vi "Main modul map v3.vi"() -> ()   [LabVIEW 2012]
uses:
  <vilib>/Utility/miscctls.llb/LVPoint32TypeDef.ctl
  <vilib>/addons/Fuzzy Logic/FL Fuzzy Controller (MIMO).vi
  Matematyczne/Matematyczne.lvlib
  <vilib>/addons/Fuzzy Logic/NI_Fuzzy_Logic_API.lvlib
panel:
  out "String":string
  in  "zad. promien odlegl.":dbl
  in  "Autonomia":bool
  out "Azymut [stopnie]":dbl
  out "Lista współrzędnych":string[][](table)
  in  "Ostatni zaznaczony punkt na mapie":cluster{"X":i32, "Y":i32}
  in  "Pocz. poł. \nrobota":T1={"UTM"={"E [m]"=393271.81, "N [m]"=5734673.27, "Strefa"=""}, "Poł. startowe"={"Piksel x"=0, "Piksel y"=0}} caption="Początkowe położenie robota" {"UTM"."N [m]" format="%#_10g"}
  in  "Tab Control":T2(tab)
  in  "Tryb GPS / Kin":u16(ring) caption="Dane na podstawie których ma działać mapa" items=["Współrzędne geografczne", "Kinematyka robota"]
  in  "Azymut robota":dbl
  in  "Lokalizacja mapy terenu":path=path "C:/Users/User/Desktop/pł.JPG"
  in  "Parametry odwzorowania Ziemi (WGS84)":cluster{"a":dbl, "b":dbl}={"a"=6378137.0, "b"=6356752.3142} {"b" format="%#.6g"; "a" format="%#.6g"}
  in  "Współrzędne geograficzne 2":string
  in  "Wyznaczanie odległości":T3(ring)=enum."Odległość pomiędzy znacznikami"
  in  "Współrzędne geograficzne 1":string
  in  "Blokada \nznaczników":bool
  in  "Zatwierdz ustalony zakres":bool
  in  "Kolor  znaczników":u32(colorbox)=16774930
  in  "Polozenie 2":cluster{"X":i32, "Y":i32}={"X"=358, "Y"=265}
  in  "Polozenie 1":cluster{"X":i32, "Y":i32}={"X"=265, "Y"=265}
  in  "Położenie na mapie":bool
  in  "Wybór \nznacznika":bool
  in  "Zaznaczona\n odleglość [m]":dbl=15.0
  in  "Zakres skali":u16(ring)=11 items=["do 1m", "do 5m", "do 10m", "do 50m", "do 100m", "do 200m", "do 500m", "do 1km", "do 5km", "do 10km", "Dubai", "OSM 10m", "OSM 30m", "OSM 50m", "OSM 100m"]
  in  "Grubość \nznaczników":u32=2
  in  "Nazwa":string
  in  "Współrzędna punktu":string
  in  "Dodaj punkt wsp.":bool
  in  "Dodaj punkt odl.":bool
  in  "Odleglosc do\n zaznaczonego punktu [m]":cluster{"X":dbl, "Y":dbl} caption="Odleglosc do zaznaczonego punktu [m] od startu"
  in  "Nazwa zaznaczonego punktu":string
  in  "Punkt do usunięcia":u16(ring) items=[""=1, "B"=2, "B"=3, "B"=4, "B"=5, "C"=6, "D"=7]
  in  "Usuń punkt":bool
  in  "Wyczyść trasę":bool
  in  "Położenie startu":bool
  in  "Kierunek na punkt":u16(ring) items=[""=1, "B"=2, "B"=3, "B"=4, "B"=5, "C"=6, "D"=7]
  out "Położenie \nrobota  UTM":T4 {"E [m]" format="%#_10g"; "N [m]" format="%#_12g"}
  out "Szerokośc geograficzna - GPS":dbl format="%_9f"
  out "Długość geograficzna - GPS":dbl format="%_9f"
  in  "Centrowanie położenia":bool
  in  "Azymut":dbl
  out "Kierunek":picture
  in  "Początkowe położenie robota":u32(colorbox)=15663118
  in  "Trasa robota":u32(colorbox)
  in  "Kierunek ruchu robota":u32(colorbox)=15663118
  in  "Zoom mapy":sgl(slide)=1.0 scale=0.2..4.0
  in  "Układ współrzędnych":u32(colorbox)
  in  "Zaznaczony punkt":u32(colorbox)=15663118 caption="Ostatni zaznaczony punkt kursorem"
  in  "Wpisane punkty na\nliście współrzędnych":u32(colorbox)=12271
  in  "Mouse down coords":T5
  out "Mapa":picture caption="Mapa z wprowadzonym punktem"
  in  "stop":bool
  # "Ustawienia dla danych z GPS\nPodstaowe parametry Ziemi dla układu WGS84"
  # "Ustawienia dla kinematyki robota."
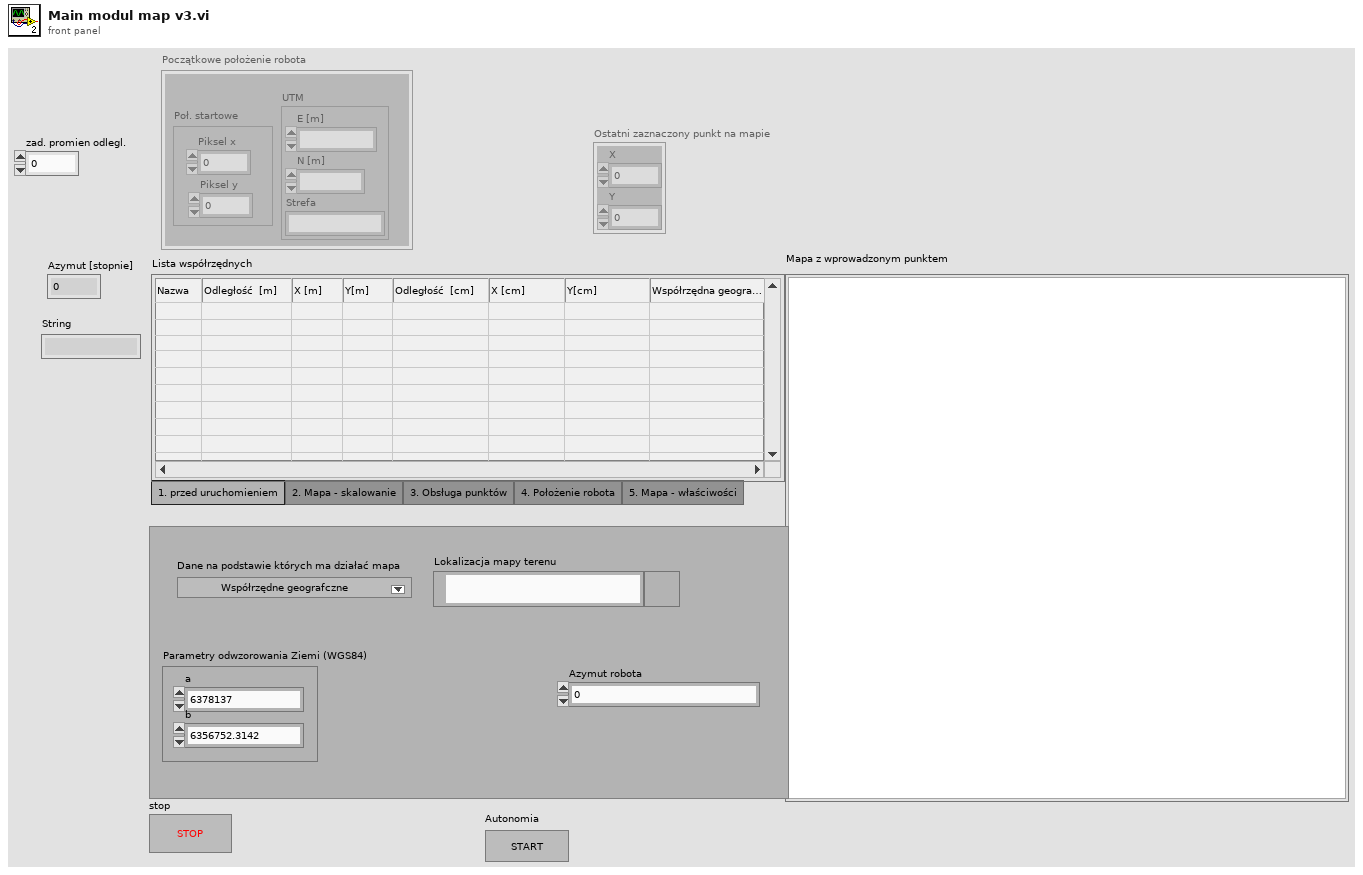
[diagram p1: front panel]
types:
  T1 = cluster{"UTM":cluster{"E [m]":ext, "N [m]":ext, "Strefa":string}, "Poł. startowe":cluster{"Piksel x":i32, "Piksel y":i32}}
  T2 = enum32{"1. przed uruchomieniem", "2. Mapa - skalowanie", "3. Obsługa punktów", "4. Położenie robota", "5. Mapa - właściwości"}
  T3 = enum16{"Współrzędne geograficzne", "Odległość pomiędzy znacznikami"}
  T4 = cluster{"E [m]":ext, "N [m]":ext, "Strefa":string}
  T5 = typedef "LVPoint32TypeDef.ctl" = cluster{"Horizontal":i32, "Vertical":i32}
  T6 = cluster{"Przesunięcie mapy":cluster{"X":i16, "Y":i16}, "Zoom":dbl, "Długość piksela w metrach":dbl}
  T7 = enum16{"Pobranie punktu", "Obrót i dojazd do punktu", "Zatrzymanie w punkcie", "Powrót na start"}
  T8 = typedef "NI_Fuzzy_Logic_API.lvlib/FL System.ctl" = cluster{"input variables":T9[], "output variables":T9[], "rules":T12[], "defuzzification method":T18, "description":string, "user MF interpolating polynomials":T19[]}
  T9 = typedef "NI_Fuzzy_Logic_API.lvlib/FL Variable.ctl" = cluster{"name":string, "range":dbl[], "MFs":T10[]}
  T10 = typedef "NI_Fuzzy_Logic_API.lvlib/FL Membership Function.ctl" = cluster{"name":string, "shape":T11, "points":dbl[], "color":u32, "user-defined shape index":i32}
  T11 = typedef "NI_Fuzzy_Logic_API.lvlib/FL Membership Function Shape.ctl" = u16
  T12 = typedef "NI_Fuzzy_Logic_API.lvlib/FL Rule.ctl" = cluster{"antecedents":T13[], "antecedent connective":T15, "consequents":T16[], "consequent implication":T17, "degree of support":dbl}
  T13 = typedef "NI_Fuzzy_Logic_API.lvlib/FL Antecedent.ctl" = cluster{"Var Index":i32, "MF Index":i32, "Cond":T14}
  T14 = typedef "NI_Fuzzy_Logic_API.lvlib/FL Modifier.ctl" = u16
  T15 = typedef "NI_Fuzzy_Logic_API.lvlib/FL Antecedent Connective.ctl" = u16
  T16 = typedef "NI_Fuzzy_Logic_API.lvlib/FL Consequent.ctl" = cluster{"Var Index":i32, "MF Index":i32, "Cond":T14}
  T17 = typedef "NI_Fuzzy_Logic_API.lvlib/FL Consequent Implication.ctl" = u16
  T18 = typedef "NI_Fuzzy_Logic_API.lvlib/FL Defuzzification.ctl" = u16
  T19 = typedef "NI_Fuzzy_Logic_API.lvlib/FL Interpolating polynomials.ctl" = cluster{"X":dbl[], "Y":dbl[], "Y(x) coeff":dbl[][], "X(y) coeff":dbl[][], "Area(y) coeff":dbl[][], "coa_x(y) coeff":dbl[][]}
  T20 = cluster{"Położenie grotu":cluster{"Pixel x":i16, "Pixel y":i16}, "Kolor":u32, "Długość [px]":u32, "Kąt/azymut":dbl, "Interpretacją kąta ustawienia strzałki":enum16{"Kąt trygonometryczny", "Azymut"}, "Grubość":u32, "Długość grotu":u32}
  T21 = cluster{"Położenie  środka":cluster{"Pixel x":i16, "Pixel y":i16}, "Kolor ":u32, "Grubość  ":u32}
  T22 = cluster{"Położenie":cluster{"Pixel x":i16, "Pixel y":i16}, "Kolor punktu":u32, "Rozmiar punktu":u32, "Nazwa punktu":string}
  T23 = cluster{"Kolor punktów z listy":u32, "Położenie startowe robota":cluster{"Pixel y":i16, "Pixel x":i16}}
  T24 = cluster{"Kolor skali":u32, "Odległość siatki od startu":cluster{"X [m]":dbl, "Y [m]":dbl}, "Poł. startowe":cluster{"Piksel x":i32, "Piksel y":i32}}
  T25 = cluster{"Nazwa zaznaczonego punktu":string, "Odleglosc do\n zaznaczonego punktu [m]":cluster{"X":dbl, "Y":dbl}}
  T26 = cluster{"UTM":cluster{"E_coord[m]":ext, "N_coord[m]":ext, "Strefa":string}, "Poł. startowe":cluster{"Piksel x":i32, "Piksel y":i32}}
  T27 = typedef "LVBoundsTypeDef.ctl" = cluster{"Width":u32, "Height":u32}
  T28 = typedef "LVMouseTypeDef.ctl" = cluster{"Mouse Position":cluster{"X":i32, "Y":i32}, "Mouse Modifiers":cluster{"Button Down":bool, "Shift Mod":bool, "Menu Mod":bool, "Option Mod":bool}}
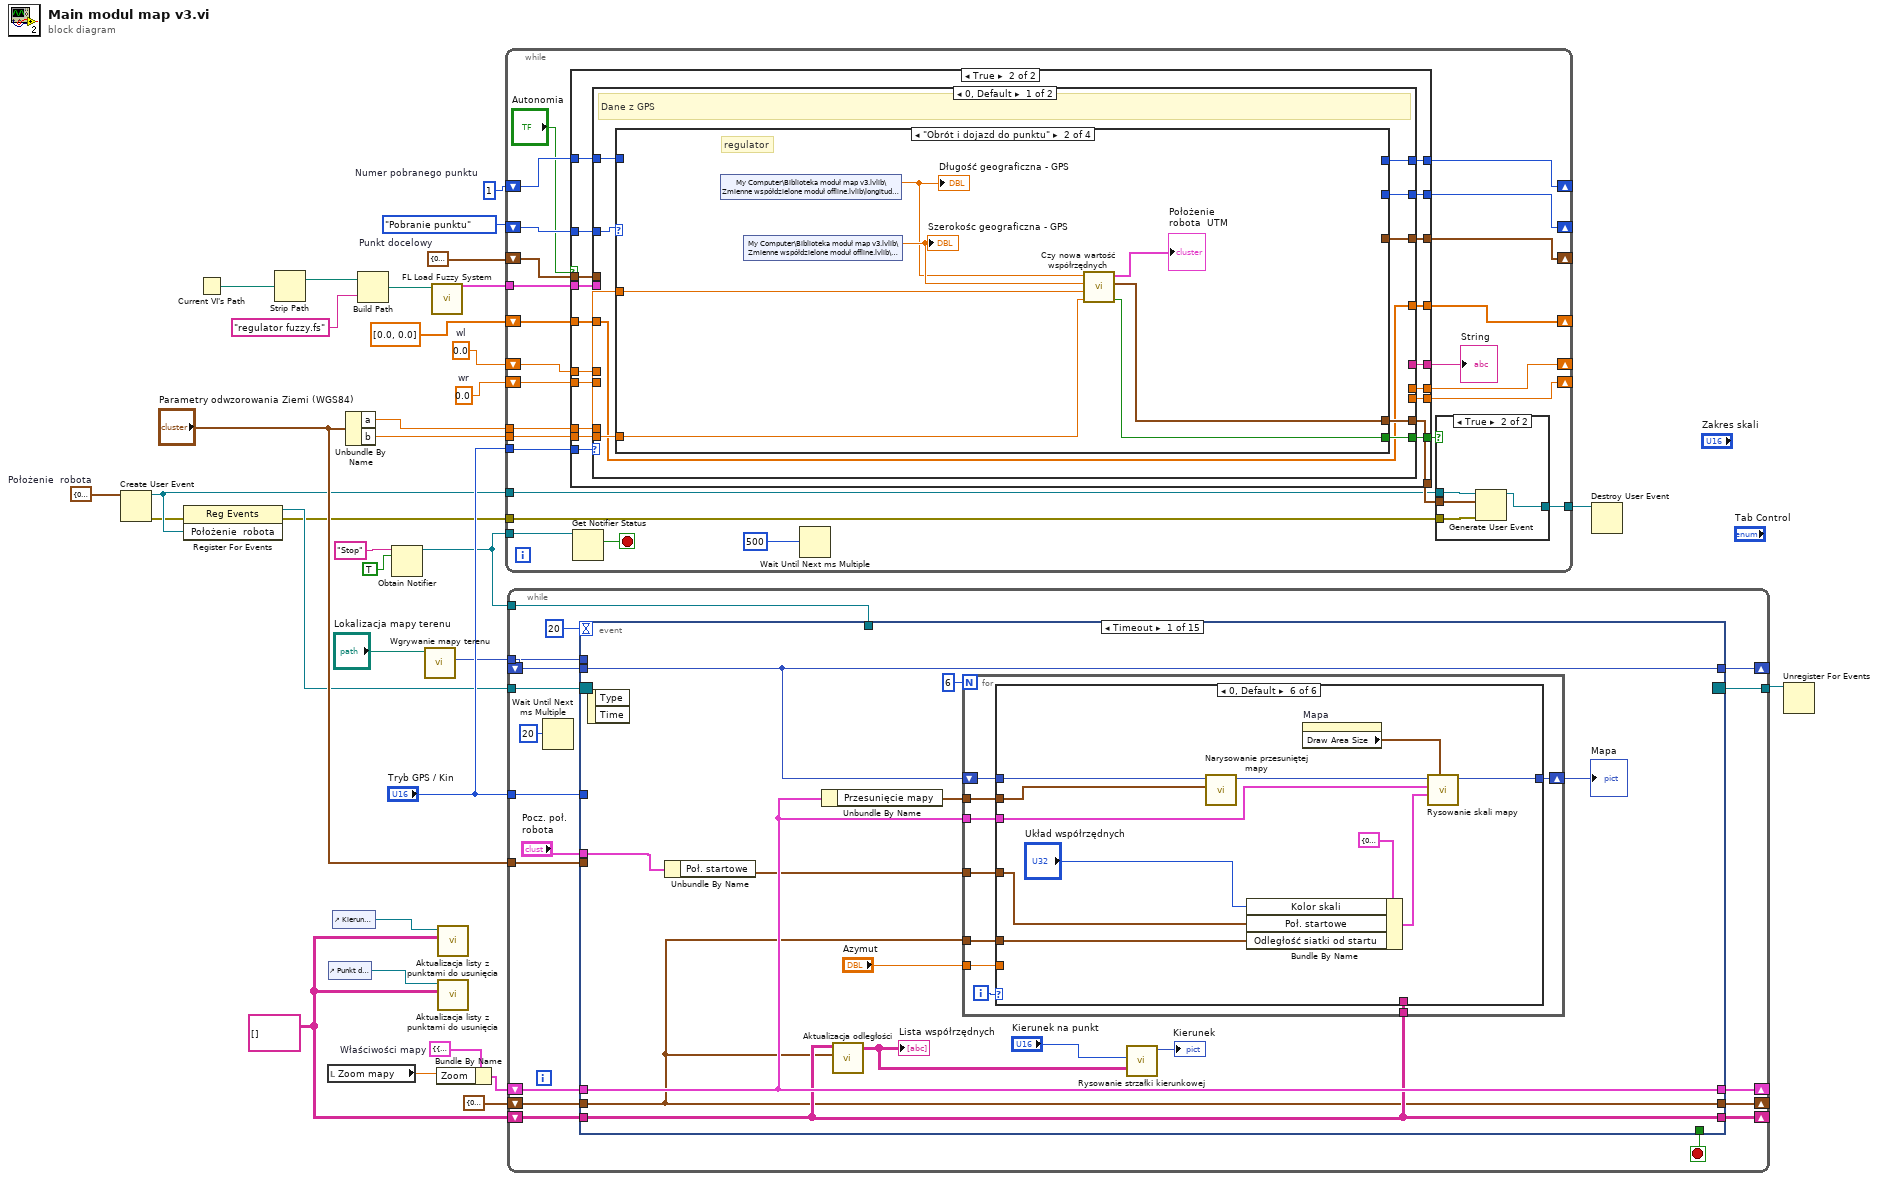
[diagram p0: block diagram]
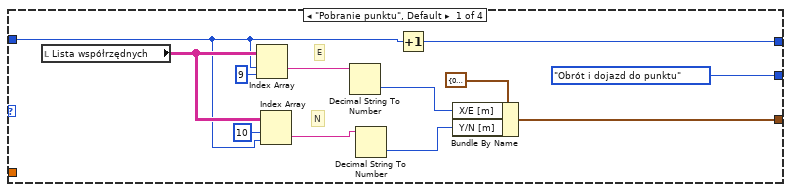
[diagram p3: hidden frame]
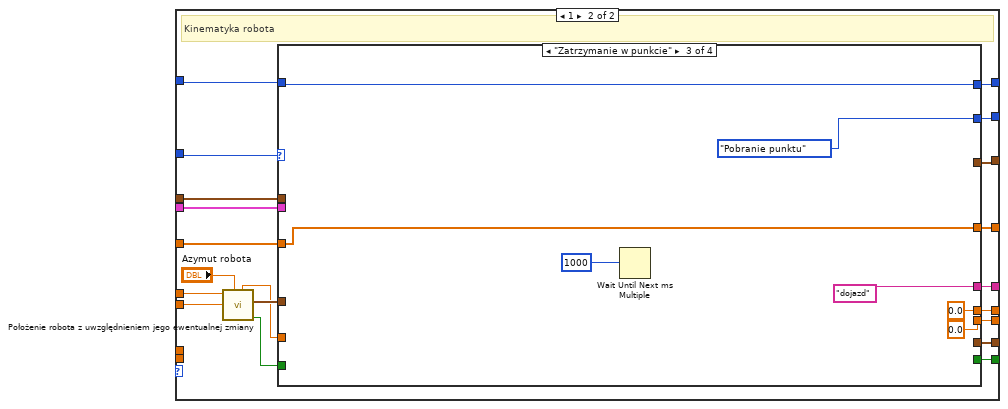
[diagram p6: hidden frame]
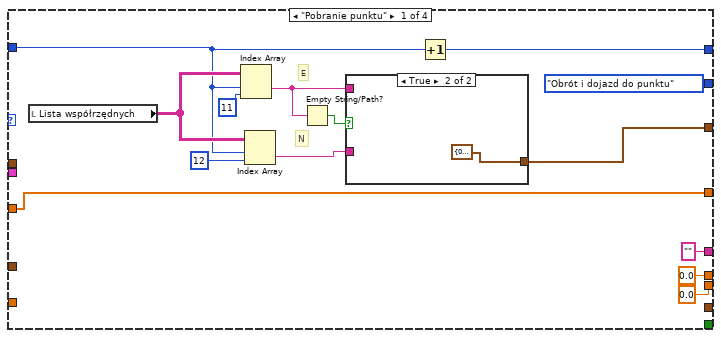
[diagram p7: hidden frame]
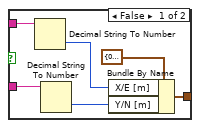
[diagram p8: hidden frame]
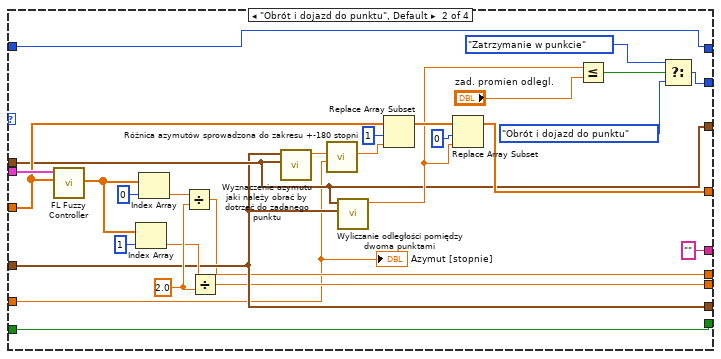
[diagram p9: hidden frame]
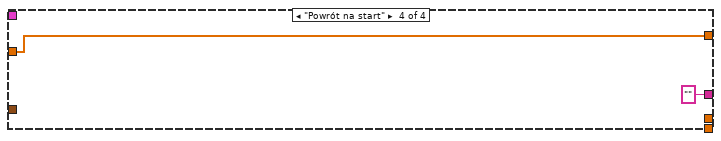
[diagram p10: hidden frame]
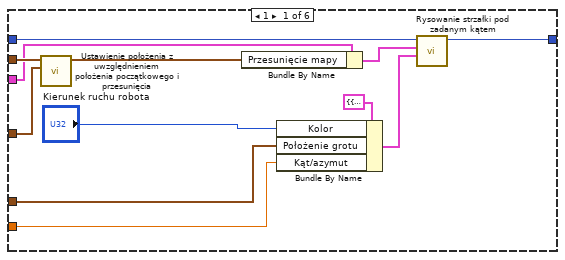
[diagram p12: hidden frame]
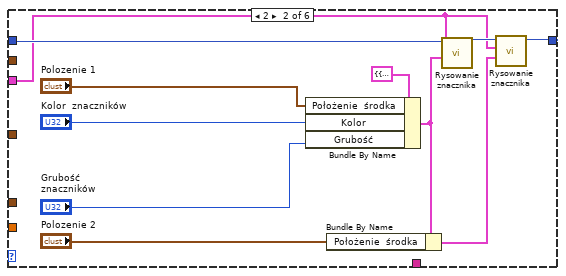
[diagram p13: hidden frame]
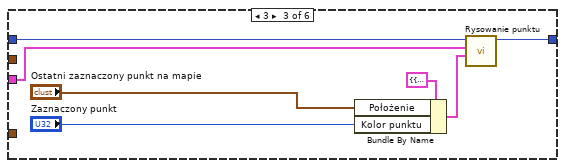
[diagram p14: hidden frame]
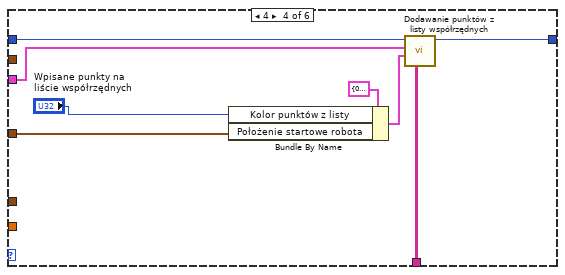
[diagram p15: hidden frame]
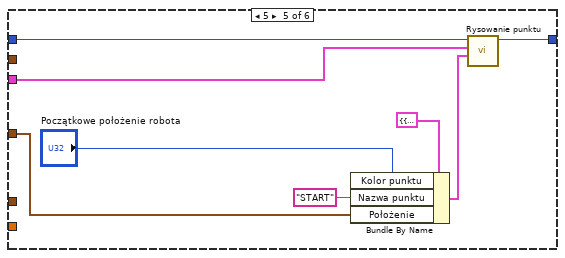
[diagram p16: hidden frame]
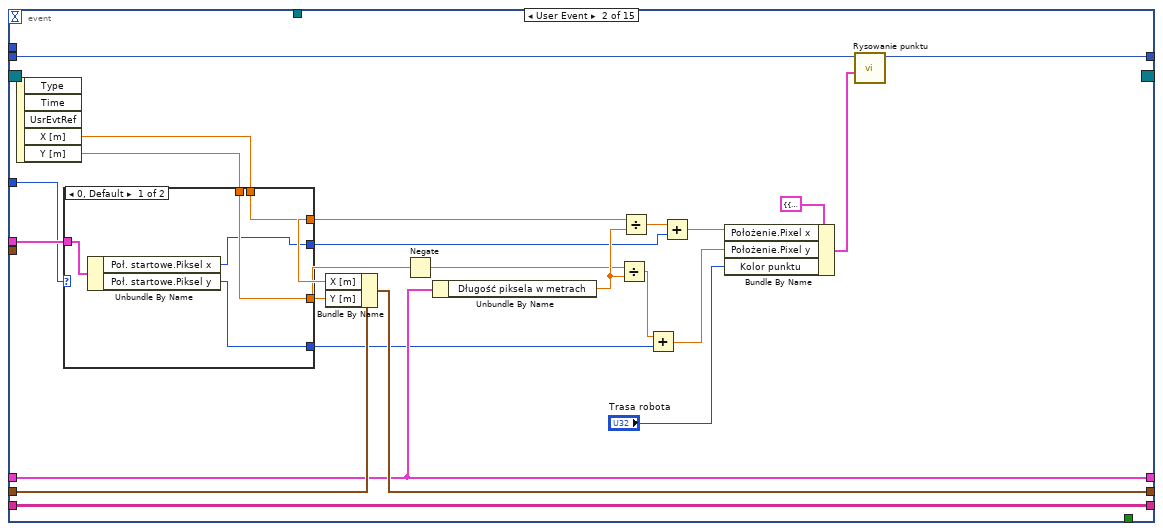
[diagram p17: hidden frame]
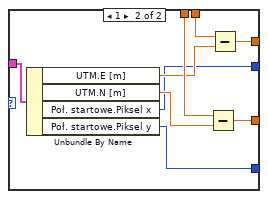
[diagram p18: hidden frame]
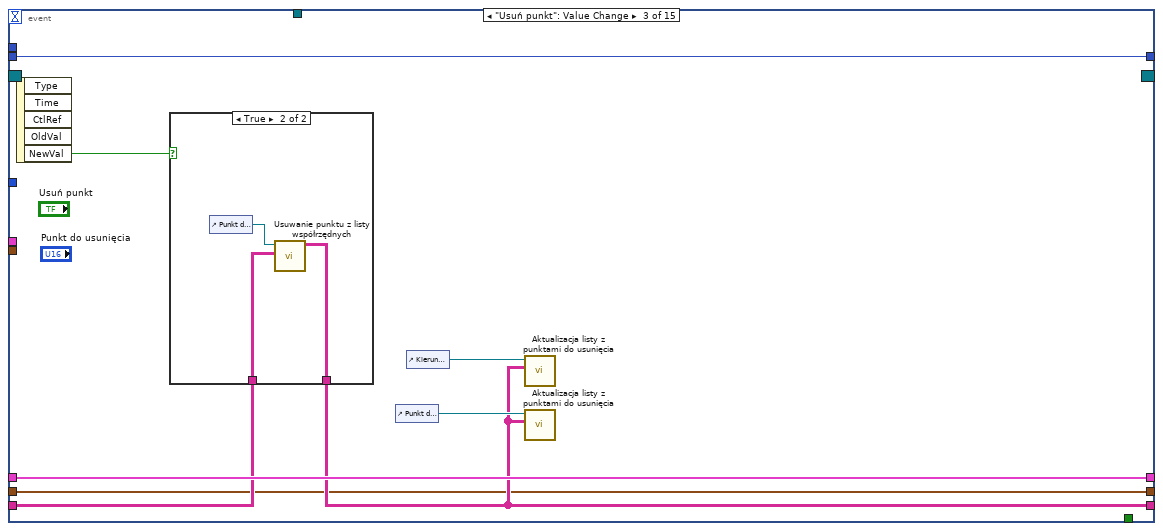
[diagram p19: hidden frame]
diagram:
  w4 = T6 {"Przesunięcie mapy"={"X"=0, "Y"=0}, "Zoom"=1.0, "Długość piksela w metrach"=0.19634281539316645}  # Właściwości mapy
  w33 = string[][] [] ("Lista współrzędnych")
  w7 = 0.0  # wr
  w8 = 0.0  # wl
  w9 = cluster{"X/E [m]":dbl, "Y/N [m]":dbl} {"X/E [m]"=0.0, "Y/N [m]"=0.0}  # Punkt docelowy
  w10 = 1  # Numer pobranego punktu
  w23 = cluster{"X [m]":dbl, "Y [m]":dbl} {"X [m]"=0.0, "Y [m]"=0.0}  # Położenie  robota
  n1 = Create User Event(user event datatype=w23) -> (user event=w21:refnum<user-event>, error out=w20:errorcluster)  [unwired: 1 in]
  n2 = register-events(error in=w20, w21) -> (reference out=w22:refnum<event-registration>)  [unwired: 1 in, 1 out]
  n3 = Current VI's Path() -> (path=w16:path)
  n4 = Strip Path(path=w16) -> (stripped path=w14:path)  [unwired: 1 out]
  n5 = local read "Zoom mapy"() -> (w1:sgl)
  n6 = control-ref of="Punkt do usunięcia"() -> (w2:refnum<vi>)
  n7 = control-ref of="Kierunek na punkt"() -> (w3:refnum<vi>)
  n8 = Unbundle By Name("Parametry odwzorowania Ziemi (WGS84)") -> ("a"=w29:dbl, "b"=w28:dbl)
  n9 = Build Path(base path=w14, name or relative path="regulator fuzzy.fs") -> (appended path=w13:path)
  n10 = Obtain Notifier(name (unnamed)="Stop", notification data type=TRUE ("create if not found? (T)")) -> (notifier out=w24:refnum<notifier>)  [unwired: 2 in, 2 out]
  n11 = call "Wgrywanie mapy terenu.vi"("Lokalizacja mapy terenu"="Lokalizacja mapy terenu") -> ("Mapa terenu"=w17:picture)  [unwired: 10 in]
  n12 = call <vilib>:"FL Load Fuzzy System.vi"("file path"=w13) -> ("fuzzy system out"=w12:T8)  [unwired: 1 in, 9 out]
  n13 = Bundle By Name(cluster=w4, "Zoom"=w1) -> (w32:T6)
  n14 = call "Aktualizacja listy z punktami do usunięcia.vi"("Lista współrzędnych"=w33, "Lista z punktami do usunięcia"=w3) -> ()  [unwired: 10 in]
  n15 = call "Aktualizacja listy z punktami do usunięcia.vi"("Lista współrzędnych"=w33, "Lista z punktami do usunięcia"=w2) -> ()  [unwired: 10 in]
  n16 = while {
    tunnel: w29 -> [w59]
    tunnel: w28 -> [w58]
    tunnel: "Tryb GPS / Kin" -> [w57]
    tunnel: w24 -> [w56]
    tunnel: w21 -> [w51]
    tunnel: w20 -> [w50]
    tunnel: [w49] -> w18
    tunnel: w12 -> [w48]
    shift-right: [w46] -> _
    shift-left: dbl[] [0.0, 0.0] ("input values") -> [w47]
    shift-right: [w42] -> _
    shift-left: T7."Pobranie punktu" -> [w45]
    shift-right: [w43] -> _
    shift-left: w10 -> [w44]
    shift-right: [w41] -> _
    shift-left: w9 -> [w40]
    shift-right: [w35] -> _
    shift-left: w8 -> [w37]
    shift-right: [w34] -> _
    shift-left: w7 -> [w36]
    stop <- w55 stop-if-true
    n17 = case shown="True" "Autonomia" {
      tunnel: w59 -> [_ w79]
      tunnel: w58 -> [_ w78]
      tunnel: w57 -> [_ w77]
      tunnel: [_ w76] -> w53
      tunnel: [_ w75] -> w52
      tunnel: w48 -> [_ w74]
      tunnel: w47 -> [w60 w73]
      tunnel: [w60 w72] -> w46
      tunnel: w45 -> [_ w71]
      tunnel: w44 -> [_ w70]
      tunnel: [_ w69] -> w43
      tunnel: [_ w68] -> w42
      tunnel: [_ w67] -> w41
      tunnel: w40 -> [_ w66]
      tunnel: [_ w65] -> w38
      tunnel: w37 -> [_ w64]
      tunnel: w36 -> [_ w63]
      tunnel: [_ w62] -> w35
      tunnel: [_ w61] -> w34
      frame False {
      }
      frame True {
        n18 = case shown="0, Default" w77 {
          tunnel: [w82 w128] -> w75
          tunnel: [w81 w127] -> w76
          tunnel: w79 -> [w84 _]
          tunnel: w78 -> [w83 _]
          tunnel: w74 -> [_ w126]
          tunnel: w73 -> [w80 w125]
          tunnel: [w80 w124] -> w72
          tunnel: w71 -> [w89 w123]
          tunnel: w70 -> [w88 w122]
          tunnel: [w87 w121] -> w69
          tunnel: [w86 w120] -> w68
          tunnel: [w85 w119] -> w67
          tunnel: w66 -> [_ w118]
          tunnel: [_ w117] -> w65
          tunnel: w64 -> [_ w115]
          tunnel: w63 -> [_ w114]
          tunnel: [_ w110] -> w62
          tunnel: [_ w109] -> w61
          frame 0, Default {
            # "Dane z GPS"
            n19 = case shown="\"Obrót i dojazd do punktu\"" w89 {
              tunnel: w88 -> [w98 _ _ _]
              tunnel: [w97 _ _ _] -> w87
              tunnel: [T7."Obrót i dojazd do punktu" _ _ _] -> w86
              tunnel: [w90 _ _ _] -> w85
              tunnel: w84 -> [_ w105 _ _]
              tunnel: w83 -> [_ w104 _ _]
              tunnel: [_ w103 _ _] -> w82
              tunnel: [_ w102 _ _] -> w81
              frame "Pobranie punktu", Default {
                # "N"
                # "E"
                n20 = local read "Lista współrzędnych"() -> (w101:string[][])
                n21 = Index Array(array=w101, index (row)=w98, index (col)=9 ("disabled index (col)")) -> (element=w96:string)
                n22 = Index Array(array=w101, index (row)=10, index (col)=w98) -> (element=w95:string)
                n23 = Decimal String To Number(string=w96) -> (number=w93:i32)  [unwired: 2 in, 1 out]
                n24 = Decimal String To Number(string=w95) -> (number=w92:i32)  [unwired: 2 in, 1 out]
                n25 = Increment(x=w98) -> (x+1=w97:i32)
                n26 = Bundle By Name(cluster=cluster{"X/E [m]":dbl, "Y/N [m]":dbl} {"X/E [m]"=0.0, "Y/N [m]"=0.0} ("Położenie"), "X/E [m]"=w93, "Y/N [m]"=w92) -> (w90:cluster{"X/E [m]":dbl, "Y/N [m]":dbl})
              }
              frame "Obrót i dojazd do punktu" {
                # "regulator"
                n27 = shared-variable "My Computer\\Biblioteka moduł map v3.lvlib\\Zmienne współdzielone moduł offline.lvlib\\longitude.longitude (deg)"() -> (w107:dbl)  [unwired: 1 in, 1 out]
                "Długość geograficzna - GPS" <- w107
                n28 = shared-variable "My Computer\\Biblioteka moduł map v3.lvlib\\Zmienne współdzielone moduł offline.lvlib\\latitude.latitude (deg)"() -> (w108:dbl)  [unwired: 1 in, 1 out]
                "Szerokośc geograficzna - GPS" <- w108
                n29 = call "Czy nowa wartość współrzędnych.vi"("b"=w104, "a"=w105, "szerokość geograficzna"=w108, "Długość geograficzna"=w107) -> ("Czy nowa wartość"=w102:bool, "Położenie"=w103:cluster{"X/E [m]":dbl, "Y/N [m]":dbl}, "Położenie \nrobota  UTM"=→"Położenie \nrobota  UTM":T4)  [unwired: 5 in]
              }
              frame "Zatrzymanie w punkcie" {
              }
              frame "Powrót na start" {
              }
            }
          }
          frame 1 {
            # "Kinematyka robota"
            n30 = call "Położenie robota z uwzględnieniem jego ewentualnej zmiany.vi"("Azymut robota"="Azymut robota", "Prędkość kątowa prawych kół [rad/s]"=w114, "Prędkość kątowa lewych kół [rad/s]"=w115) -> ("Boolean"=w111:bool, "Cluster"=w113:cluster{"X [m]":dbl, "Y [m]":dbl}, "Azymut [stopnie]"=w112:dbl)  [unwired: 6 in]
            n31 = case shown="\"Zatrzymanie w punkcie\"" w123 {
              tunnel: [_ w157 _ _] -> w128
              tunnel: [_ w156 _ _] -> w127
              tunnel: w126 -> [_ w177 _ _]
              tunnel: w125 -> [w131 w176 w178 w185]
              tunnel: [w131 w175 w178 w185] -> w124
              tunnel: w122 -> [w135 w153 w181 _]
              tunnel: [w139 w153 w181 _] -> w121
              tunnel: [T7."Obrót i dojazd do punktu" w160 T7."Pobranie punktu" _] -> w120
              tunnel: [w137 w159 _ _] -> w119
              tunnel: w118 -> [_ w159 _ _]
              tunnel: ["" "" "dojazd" ""] -> w117
              tunnel: w113 -> [_ w157 _ _]
              tunnel: w112 -> [_ w150 _ _]
              tunnel: w111 -> [_ w156 _ _]
              tunnel: [0.0 w155 0.0 _] -> w110
              tunnel: [0.0 w154 0.0 _] -> w109
              frame "Pobranie punktu" {
                # "N"
                # "E"
                n32 = local read "Lista współrzędnych"() -> (w142:string[][])
                n33 = Index Array(array=w142, index (row)=w135, index (col)=11 ("disabled index (col)")) -> (element=w130:string)
                n34 = Index Array(array=w142, index (row)=w135, index (col)=12 ("index (row)")) -> (element=w140:string)
                n35 = Empty String/Path?(string/path=w130) -> (empty?=w129:bool)
                n36 = case shown="True" w129 {
                  tunnel: w130 -> [w148 _]
                  tunnel: w140 -> [w147 _]
                  tunnel: [w144 cluster{"X/E [m]":dbl, "Y/N [m]":dbl} {"X/E [m]"=0.0, "Y/N [m]"=0.0} ("Położenie")] -> w137
                  frame False {
                    n37 = Decimal String To Number(string=w148) -> (number=w145:i32)  [unwired: 2 in, 1 out]
                    n38 = Decimal String To Number(string=w147) -> (number=w143:i32)  [unwired: 2 in, 1 out]
                    n39 = Bundle By Name(cluster=cluster{"X/E [m]":dbl, "Y/N [m]":dbl} {"X/E [m]"=0.0, "Y/N [m]"=0.0} ("Położenie"), "X/E [m]"=w145, "Y/N [m]"=w143) -> (w144:cluster{"X/E [m]":dbl, "Y/N [m]":dbl})
                  }
                  frame True {
                  }
                }
                n40 = Increment(x=w135) -> (x+1=w139:i32)
              }
              frame "Obrót i dojazd do punktu", Default {
                w174 = 2.0 ("y")
                n41 = call-poly <vilib>:"FL Fuzzy Controller.vi"("input values"=w176, "fuzzy system in"=w177) -> ("output values"=w169:dbl[])  [unwired: 5 in, 4 out]
                n42 = Index Array(array=w169, index=1) -> (element=w172:dbl)
                n43 = Index Array(array=w169, index=0) -> (element=w173:dbl)
                n44 = Divide(x=w173, y=w174) -> (x/y=w155:dbl)
                n45 = Divide(x=w172, y=w174) -> (x/y=w154:dbl)
                n46 = call "Wyznaczenie azymutu jaki należy obrać by dotrzeć do zadanego punktu.vi"("Położenie końcowe"=w159, "Położenie aktualne"=w157) -> ("Azymut"=w151:dbl)  [unwired: 9 in]
                n47 = call "Różnica azymutów sprowadzona do zakresu +-180 stopni.vi"("Azymut robota"=w150, "Azymut - zadany"=w151) -> ("az_z - az_r"=w152:dbl)  [unwired: 9 in]
                n48 = call "Wyliczanie odległości pomiędzy dwoma punktami.vi"("Polozenie 1"=w157, "Polozenie in"=w159) -> ("Numeric"=w165:dbl)  [unwired: 9 in]
                n49 = Replace Array Subset(array=w176, new element=w152, index=1) -> (w167:dbl[])
                n50 = Replace Array Subset(array=w167, new element=w165, index=0) -> (w175:dbl[])
                n51 = Less Or Equal?(x=w165, y="zad. promien odlegl.") -> (x <= y?=w163:bool)
                n52 = Select(t=T7."Zatrzymanie w punkcie", s=w163, f=T7."Obrót i dojazd do punktu") -> (s? t:f=w160:T7)
                "Azymut [stopnie]" <- w150
              }
              frame "Zatrzymanie w punkcie" {
                n53 = Wait Until Next ms Multiple(millisecond multiple=u32 1000) -> ()  [unwired: 1 out]
              }
              frame "Powrót na start" {
              }
            }
          }
        }
      }
    }
    "String" <- w38
    n54 = Get Notifier Status(notifier=w56) -> (current notification=w55:bool)  [unwired: 1 in, 4 out]
    n55 = Wait Until Next ms Multiple(millisecond multiple=u32 500) -> ()  [unwired: 1 out]
    n56 = case shown="True" w53 {
      tunnel: w52 -> [_ w191]
      tunnel: w51 -> [w187 w190]
      tunnel: w50 -> [_ w189]
      tunnel: [w187 w188] -> w49
      frame False {
      }
      frame True {
        n57 = Generate User Event(user event=w190, event data cluster=w191, error in=w189) -> (user event out=w188:refnum<user-event>)  [unwired: 1 out]
      }
    }
  }
  n58 = while {
    shift-right: [w209] -> _
    shift-left: w32 -> [w208]
    shift-right: [w204] -> _
    shift-left: w17 -> [w205]
    shift-right: [w202] -> _
    shift-left: w33 -> [w203]
    tunnel: "Parametry odwzorowania Ziemi (WGS84)" -> [w201]
    shift-right: [w200] -> _
    shift-left: cluster{"X [m]":dbl, "Y [m]":dbl} {"X [m]"=0.0, "Y [m]"=0.0} ("Odległość od startu [m]") -> [w199]
    tunnel: w24 -> [w198]
    tunnel: "Tryb GPS / Kin" -> [w192]
    tunnel: w22 -> [w197]
    tunnel: [w196] -> w19
    tunnel: w17 -> [w194]
    stop <- w207 stop-if-true
    n59 = Wait Until Next ms Multiple(millisecond multiple=u32 20) -> ()  [unwired: 1 out]
    n60 = event shown="[0] Timeout" {
      selector: w197 -> [_ _ _ _ _ _ _ _ _ _ _ _ _ _ _]
      dyn-events: [_ _ _ _ _ _ _ _ _ _ _ _ _ _ _] -> w196
      timeout: 20 -> [_ _ _ _ _ _ _ _ _ _ _ _ _ _ _]
      tunnel: [w216 w301 w333 w350 w354 w370 w375 w381 w425 w436 w444 w447 w462 w495 w511] -> w209
      tunnel: w208 -> [w216 w301 w333 w350 w355 w370 w375 w384 w424 w434 w444 w447 w461 w495 w511]
      tunnel: w205 -> [w222 w305 w332 w349 _ _ w374 w392 w429 _ w443 w451 w480 w500 w510]
      tunnel: [_ _ _ _ _ _ _ _ _ _ "stop" _ _ _ _] -> w207
      tunnel: [w222 w306 w332 w349 w351 w367 w374 w392 w429 w430 w443 w451 w480 w500 w510] -> w204
      tunnel: w203 -> [w214 w311 w330 w348 w357 w369 w372 w385 w427 w438 w442 w448 w478 w499 w509]
      tunnel: [w214 w311 w327 w339 w357 w369 w372 w385 w427 w438 w442 w448 w478 w499 w502] -> w202
      tunnel: w201 -> [_ _ _ w342 _ _ _ w383 _ _ _ _ _ _ _]
      tunnel: [w211 w308 w326 w338 w352 w368 w371 cluster{"X [m]":dbl, "Y [m]":dbl} {"X [m]"=0.0, "Y [m]"=0.0} ("Odległość od startu [m]") w420 w437 w441 w445 w459 w483 w501] -> w200
      tunnel: w199 -> [w211 w309 w326 w338 w352 w368 w371 _ w420 w437 w441 w445 w459 w483 w501]
      tunnel: w198 -> [_ _ _ _ _ _ _ _ _ _ w440 _ _ _ _]
      tunnel: "Pocz. poł. \nrobota" -> [w210 w310 _ _ _ _ _ _ w419 w435 _ _ _ _ _]
      tunnel: w194 -> [_ _ _ _ w351 w367 _ _ _ w430 _ _ _ _ _]
      tunnel: w192 -> [_ w289 _ _ _ _ _ w382 _ _ _ _ _ _ _]
      event Timeout {
        n61 = event-data() -> ()  [unwired: 1 in, 2 out]
        n62 = Unbundle By Name(w210) -> ("Poł. startowe"=w212:cluster{"Piksel x":i32, "Piksel y":i32})
        n63 = Unbundle By Name(w216) -> ("Przesunięcie mapy"=w219:cluster{"X":i16, "Y":i16})
        n64 = call "Aktualizacja odległości.vi"("Odległość od startu [m]"=w211, "Lista współrzędnych"=w214) -> ("Lista współrzędnych 2"=w213:string[][])  [unwired: 9 in]
        "Lista współrzędnych" <- w213
        n65 = for {
          N: 6 -> [_]
          shift-right: [w230] -> w221
          shift-left: w222 -> [w231]
          tunnel: w211 -> [w229]
          tunnel: w214 -> [w227]
          tunnel: w212 -> [w226]
          tunnel: w219 -> [w225]
          tunnel: w216 -> [w224]
          tunnel: "Azymut" -> [w223]
          i -> [w228]
          n66 = case shown="0, Default" w228 {
            tunnel: w225 -> [w237 _ _ _ _ w283]
            tunnel: w231 -> [w242 w246 w257 w269 w277 w285]
            tunnel: [w243 w245 w258 w268 w273 w284] -> w230
            tunnel: w229 -> [w232 _ _ _ _ w278]
            tunnel: w227 -> [_ _ _ w267 _ _]
            tunnel: w226 -> [w238 _ _ w262 w270 w279]
            tunnel: w224 -> [w234 w244 w255 w263 w272 w282]
            tunnel: w223 -> [w233 _ _ _ _ _]
            frame 1 {
              n67 = call "Ustawienie położenia z uwzględnieniem położenia początkowego i przesunięcia.vi"("Poł. startowe"=w238, "Przesunięcie mapy"=w237) -> ("Początkowe położenie robota out"=w235:cluster{"X":i16, "Y":i16})  [unwired: 9 in]
              n68 = Bundle By Name(cluster=w234, "Przesunięcie mapy"=w235) -> (w236:T6)
              n69 = Bundle By Name(cluster=T20 {"Położenie grotu"={"Pixel x"=0, "Pixel y"=0}, "Kolor"=0, "Długość [px]"=26, "Kąt/azymut"=2.0, "Interpretacją kąta ustawienia strzałki"=enum."Azymut", "Grubość"=2, "Długość grotu"=10} ("Parametry strzałki"), "Kolor"="Kierunek ruchu robota", "Położenie grotu"=w232, "Kąt/azymut"=w233) -> (w239:T20)
              n70 = call "Rysowanie strzałki pod zadanym kątem.vi"("Parametry strzałki"=w239, "Właściwości mapy"=w236, "Mapa terenu"=w242) -> ("Mapa ze strzałką"=w243:picture)  [unwired: 8 in]
            }
            frame 2 {
              n71 = Bundle By Name(cluster=T21 {"Położenie  środka"={"Pixel x"=0, "Pixel y"=0}, "Kolor "=0, "Grubość  "=3} ("Znacznik na mapie"), "Położenie  środka"="Polozenie 1", "Kolor"="Kolor  znaczników", "Grubość"="Grubość \nznaczników") -> (w251:T21)
              n72 = Bundle By Name(cluster=w251, "Położenie  środka"="Polozenie 2") -> (w252:T21)
              n73 = call "Rysowanie znacznika.vi"("Znacznik na mapie"=w251, "Właściwości mapy"=w244, "Mapa terenu"=w246) -> ("Mapa z wprowadzonym znacznikiem"=w247:picture)  [unwired: 8 in]
              n74 = call "Rysowanie znacznika.vi"("Znacznik na mapie"=w252, "Właściwości mapy"=w244, "Mapa terenu"=w247) -> ("Mapa z wprowadzonym znacznikiem"=w245:picture)  [unwired: 8 in]
            }
            frame 3 {
              n75 = Bundle By Name(cluster=T22 {"Położenie"={"Pixel x"=0, "Pixel y"=0}, "Kolor punktu"=0, "Rozmiar punktu"=2, "Nazwa punktu"=""} ("Punkt na mapie"), "Położenie"="Ostatni zaznaczony punkt na mapie", "Kolor punktu"="Zaznaczony punkt") -> (w260:T22)
              n76 = call "Rysowanie punktu.vi"("Punkt na mapie"=w260, "Właściwości mapy"=w255, "Mapa terenu"=w257) -> ("Mapa z wprowadzonym punktem"=w258:picture)  [unwired: 8 in]
            }
            frame 4 {
              n77 = Bundle By Name(cluster=T23 {"Kolor punktów z listy"=0, "Położenie startowe robota"={"Pixel y"=0, "Pixel x"=0}} ("Właściwości punktów z listy"), "Kolor punktów z listy"="Wpisane punkty na\nliście współrzędnych", "Położenie startowe robota"=w262) -> (w264:T23)
              n78 = call "Dodawanie punktów z listy współrzędnych.vi"("Lista współrzędnych"=w267, "Właściwości punktów z listy"=w264, "Właściwości mapy"=w263, "Mapa terenu"=w269) -> ("Mapa z wprowadzonym punktem"=w268:picture)  [unwired: 7 in]
            }
            frame 5 {
              n79 = Bundle By Name(cluster=T22 {"Położenie"={"Pixel x"=0, "Pixel y"=0}, "Kolor punktu"=0, "Rozmiar punktu"=2, "Nazwa punktu"=""} ("Punkt na mapie"), "Kolor punktu"="Początkowe położenie robota", "Nazwa punktu"="START", "Położenie"=w270) -> (w275:T22)
              n80 = call "Rysowanie punktu.vi"("Punkt na mapie"=w275, "Właściwości mapy"=w272, "Mapa terenu"=w277) -> ("Mapa z wprowadzonym punktem"=w273:picture)  [unwired: 8 in]
            }
            frame 0, Default {
              n81 = call "Narysowanie przesuniętej mapy.vi"("Przesunięcie mapy"=w283, "Mapa"=w285) -> ("Przesunięta mapa"=w286:picture)  [unwired: 9 in]
              n82 = Bundle By Name(cluster=T24 {"Kolor skali"=0, "Odległość siatki od startu"={"X [m]"=0.0, "Y [m]"=0.0}, "Poł. startowe"={"Piksel x"=115, "Piksel y"=101}} ("Parametry"), "Kolor skali"="Układ współrzędnych", "Poł. startowe"=w279, "Odległość siatki od startu"=w278) -> (w280:T24)
              n83 = property on="Mapa" class="Pict"() -> ("Draw Area Size"=w288:T27)  [unwired: 2 in, 2 out]
              n84 = call "Rysowanie skali mapy.vi"("Rozmiar obszaru widocznej mapy"=w288, "Parametry"=w280, "Właściwości mapy"=w282, "Obraz wejściowy"=w286) -> ("Obraz wyjściowy"=w284:picture)  [unwired: 7 in]
            }
          }
        }
        "Mapa" <- w221
        n85 = call "Rysowanie strzałki kierunkowej.vi"("Lista współrzędnych"=w213, "Kierunek na punkt in"="Kierunek na punkt") -> ("Mapa ze strzałką"=→"Kierunek":picture)  [unwired: 8 in, 1 out]
      }
      event User Event {
        n86 = event-data() -> ("X [m]"=w298:dbl, "Y [m]"=w307:dbl)  [unwired: 1 in, 3 out]
        n87 = case shown="0, Default" w289 {
          tunnel: w310 -> [w314 w325]
          tunnel: w307 -> [w315 w324]
          tunnel: [w316 w322] -> w299
          tunnel: w298 -> [w316 w321]
          tunnel: [w313 w319] -> w296
          tunnel: [w312 w318] -> w295
          tunnel: [w315 w317] -> w291
          frame 0, Default {
            n88 = Unbundle By Name(w314) -> ("Poł. startowe.Piksel x"=w313:i32, "Poł. startowe.Piksel y"=w312:i32)
          }
          frame 1 {
            n89 = Unbundle By Name(w325) -> ("UTM.E [m]"=w320:ext, "UTM.N [m]"=w323:ext, "Poł. startowe.Piksel x"=w319:i32, "Poł. startowe.Piksel y"=w318:i32)
            n90 = Subtract(x=w324, y=w323) -> (x-y=w317:ext)
            n91 = Subtract(x=w321, y=w320) -> (x-y=w322:ext)
          }
        }
        n92 = Bundle By Name(cluster=w309, "X [m]"=w299, "Y [m]"=w291) -> (w308:cluster{"X [m]":dbl, "Y [m]":dbl})
        n93 = Negate(x=w291) -> (-x=w290:ext)
        n94 = Unbundle By Name(w301) -> ("Długość piksela w metrach"=w300:dbl)
        n95 = Divide(x=w290, y=w300) -> (x/y=w294:ext)
        n96 = Divide(x=w299, y=w300) -> (x/y=w297:ext)
        n97 = Add(x=w294, y=w295) -> (x+y=w293:ext)
        n98 = Add(x=w297, y=w296) -> (x+y=w292:ext)
        n99 = Bundle By Name(cluster=T22 {"Położenie"={"Pixel x"=0, "Pixel y"=0}, "Kolor punktu"=0, "Rozmiar punktu"=2, "Nazwa punktu"=""} ("Punkt na mapie"), "Położenie.Pixel x"=w292, "Położenie.Pixel y"=w293, "Kolor punktu"="Trasa robota") -> (w303:T22)
        n100 = call "Rysowanie punktu.vi"("Punkt na mapie"=w303, "Mapa terenu"=w305) -> ("Mapa z wprowadzonym punktem"=w306:picture)  [unwired: 9 in]
      }
      event "Usuń punkt": Value Change {
        n101 = event-data() -> ("NewVal"=w331:bool)  [unwired: 1 in, 4 out]
        n102 = case shown="True" w331 {
          tunnel: w330 -> [w334 w335]
          tunnel: [w334 w337] -> w327
          frame False {
          }
          frame True {
            n103 = control-ref of="Punkt do usunięcia"() -> (w336:refnum<vi>)
            n104 = call "Usuwanie punktu z listy współrzędnych.vi"("Lista współrzędnych"=w335, "Lista z punktami do usunięcia"=w336) -> ("Lista współrzędnych 2"=w337:string[][])  [unwired: 9 in]
          }
        }
        n105 = control-ref of="Punkt do usunięcia"() -> (w328:refnum<vi>)
        n106 = control-ref of="Kierunek na punkt"() -> (w329:refnum<vi>)
        n107 = call "Aktualizacja listy z punktami do usunięcia.vi"("Lista współrzędnych"=w327, "Lista z punktami do usunięcia"=w329) -> ()  [unwired: 10 in]
        n108 = call "Aktualizacja listy z punktami do usunięcia.vi"("Lista współrzędnych"=w327, "Lista z punktami do usunięcia"=w328) -> ()  [unwired: 10 in]
      }
      event "Dodaj punkt odl.": Value Change {
        n109 = event-data() -> ()  [unwired: 1 in, 5 out]
        n110 = local read "Pocz. poł. \nrobota"() -> (w347:T1)
        n111 = Bundle By Name(cluster=T25 {"Nazwa zaznaczonego punktu"="er", "Odleglosc do\n zaznaczonego punktu [m]"={"X"=23.89186471933565, "Y"=43.80175198544869}} ("Zaznaczony punkt"), "Nazwa zaznaczonego punktu"="Nazwa zaznaczonego punktu", "Odleglosc do\n zaznaczonego punktu [m]"="Odleglosc do\n zaznaczonego punktu [m]") -> (w345:T25)
        n112 = call "Dodawanie punktu na podstawie odległości od robota w kierunku xy.vi"("Parametry odwzorowania Ziemi"=w342, "Zaznaczony punkt"=w345, "Początkowe położenie robota"=w347, "Lista współrzędnych"=w348) -> ("output array"=w339:string[][])  [unwired: 7 in]
        n113 = control-ref of="Punkt do usunięcia"() -> (w340:refnum<vi>)
        n114 = control-ref of="Kierunek na punkt"() -> (w341:refnum<vi>)
        n115 = call "Aktualizacja listy z punktami do usunięcia.vi"("Lista współrzędnych"=w339, "Lista z punktami do usunięcia"=w340) -> ()  [unwired: 10 in]
        n116 = call "Aktualizacja listy z punktami do usunięcia.vi"("Lista współrzędnych"=w339, "Lista z punktami do usunięcia"=w341) -> ()  [unwired: 10 in]
      }
      event "Zatwierdz ustalony zakres": Value Change {
        n117 = event-data() -> ()  [unwired: 1 in, 5 out]
        n118 = local read "Wyznaczanie odległości"() -> (w362:T3)
        n119 = case shown="\"Współrzędne geograficzne\", Default" w362 {
          tunnel: [w364 "Zaznaczona\n odleglość [m]"] -> w353
          frame "Współrzędne geograficzne", Default {
            n120 = call "Wyznaczanie odległości pomiędzy dwoma współrzędnymi geograficznymi.vi"("Współrzędne geograficzne in"="Współrzędne geograficzne 2", "Współrzędne geograficzne 1"="Współrzędne geograficzne 1") -> ("Numeric"=w364:dbl)  [unwired: 9 in]
          }
          frame "Odległość pomiędzy znacznikami" {
          }
        }
        n121 = local write "Blokada \nznaczników"(TRUE ("Blokada \nznaczników")) -> ()
        n122 = local read "Polozenie 2"() -> (w360:cluster{"X":i32, "Y":i32})
        n123 = local read "Polozenie 1"() -> (w361:cluster{"X":i32, "Y":i32})
        n124 = call "Wyliczanie odległości pomiędzy dwoma punktami.vi"("Polozenie 1"=w361, "Polozenie in"=w360) -> ("Numeric"=w359:dbl)  [unwired: 9 in]
        n125 = Divide(x=w353, y=w359) -> (x/y=w356:dbl)
        n126 = Bundle By Name(cluster=w355, "Długość piksela w metrach"=w356) -> (w354:T6)
      }
      event "Wyczyść trasę": Value Change {
        n127 = event-data() -> ()  [unwired: 1 in, 5 out]
      }
      event "Wyznaczanie odległości": Value Change {
        n128 = event-data() -> ()  [unwired: 1 in, 5 out]
        n129 = case shown="\"Współrzędne geograficzne\", Default" "Wyznaczanie odległości" {
          frame "Współrzędne geograficzne", Default {
            w376 = TRUE ("Visible")
            n130 = property on="Zaznaczona\n odleglość [m]" class="DigNum (strict)"("Visible"=FALSE) -> ()  [unwired: 2 in, 2 out]
            n131 = property on="Współrzędne geograficzne 1" class="Str"("Visible"=w376) -> ()  [unwired: 2 in, 2 out]
            n132 = property on="Współrzędne geograficzne 2" class="Str"("Visible"=w376) -> ()  [unwired: 2 in, 2 out]
          }
          frame "Odległość pomiędzy znacznikami" {
            w378 = FALSE ("Visible")
            n133 = property on="Zaznaczona\n odleglość [m]" class="DigNum (strict)"("Visible"=TRUE) -> ()  [unwired: 2 in, 2 out]
            n134 = property on="Współrzędne geograficzne 1" class="Str"("Visible"=w378) -> ()  [unwired: 2 in, 2 out]
            n135 = property on="Współrzędne geograficzne 2" class="Str"("Visible"=w378) -> ()  [unwired: 2 in, 2 out]
          }
        }
      }
      event "Położenie na mapie": Value Change {
        # "Ostatnie zaznaczone na mapie położenie odpowiada lokalizacji robota na mapie terenu."
        n136 = event-data() -> ()  [unwired: 1 in, 5 out]
        n137 = local read "Mouse down coords"() -> (w391:T5)
        n138 = feedback-in #1(w391) -> ()
        n139 = feedback #1() -> (w390:T5)  [unwired: 1 in]
        n140 = Not Equal?(x=w391, y=w390) -> (x != y?=w389:cluster{"Horizontal":bool, "Vertical":bool})
        n141 = Unbundle By Name(w389) -> ("Horizontal"=w387:bool, "Vertical"=w386:bool)
        n142 = Or(x=w387, y=w386) -> (x .or. y?=w388:bool)
        n143 = case shown="True" w388 {
          tunnel: w391 -> [_ w403]
          tunnel: w384 -> [_ w404]
          tunnel: [w393 w397] -> w381
          tunnel: w384 -> [w393 w396]
          tunnel: w382 -> [_ w395]
          tunnel: w383 -> [_ w394]
          frame False {
          }
          frame True {
            n144 = Unbundle By Name(w404) -> ("Przesunięcie mapy"=w402:cluster{"X":i16, "Y":i16})
            n145 = Subtract(x=w403, y=w402) -> (x-y=w399:T5)
            n146 = case shown="0, Default" w395 {
              tunnel: [w414 w417] -> w401
              tunnel: w399 -> [w413 w416]
              tunnel: w394 -> [w409 _]
              frame 0, Default {
                # "wsp. geograficzne"
                n147 = local read "Długość geograficzna - GPS"() -> (w405:dbl)
                n148 = local read "Szerokośc geograficzna - GPS"() -> (w406:dbl)
                n149 = Unbundle By Name(w409) -> ("a"=w407:dbl, "b"=w408:dbl)
                n150 = call "współrzedne geograficzne na UTM.vi"("Położenie robota - długość geograficzna"=w405, "Położenie robota - szerokość geograficzna"=w406, "a"=w407, "b"=w408) -> ("Strefa"=w412:string, "E"=w411:ext, "N"=w410:ext)  [unwired: 2 in]
                n151 = Bundle By Name(cluster=T26 {"UTM"={"E_coord[m]"=393353.78, "N_coord[m]"=5734793.92, "Strefa"="34U"}, "Poł. startowe"={"Piksel x"=115, "Piksel y"=101}} ("Początkowe położenie robota"), "Poł. startowe"=w413, "UTM.Strefa"=w412, "UTM.E_coord[m]"=w411, "UTM.N_coord[m]"=w410) -> (w414:T26)
              }
              frame 1 {
                n152 = Bundle By Name(cluster=T26 {"UTM"={"E_coord[m]"=0.0, "N_coord[m]"=0.0, "Strefa"=""}, "Poł. startowe"={"Piksel x"=115, "Piksel y"=101}} ("Początkowe położenie robota"), "Poł. startowe"=w416) -> (w417:T26)
              }
            }
            n153 = control-ref of="Mapa"() -> (w400:refnum<vi>)
            n154 = call "Centrowanie położenia.vi"("Ostatnie położenie robota"=w399, "Mapa z wprowadzonym punktem"=w400) -> ("Przesunięcie wycentrowane"=w398:T5)  [unwired: 9 in]
            n155 = Bundle By Name(cluster=w396, "Przesunięcie mapy"=w398) -> (w397:T6)
            n156 = local write "Pocz. poł. \nrobota"(w401) -> ()
          }
        }
      }
      event "Centrowanie położenia", "Zoom mapy": Value Change {
        n157 = event-data() -> ()  [unwired: 1 in, 5 out]
        n158 = Unbundle By Name(w424) -> ("Długość piksela w metrach"=w423:dbl)
        n159 = call "Ustawienie ostatniego położenia na podstawie odległości od punktu startowego.vi"("Długość piksela w metrach"=w423, "Odległość od startu [m]"=w420, "Początkowe położenie robota"=w419) -> ("Ostatnie położenie robota"=w422:cluster{"Pixel x":i16, "Pixel y":i16})  [unwired: 8 in]
        n160 = control-ref of="Mapa"() -> (w428:refnum<vi>)
        n161 = call "Centrowanie położenia.vi"("Ostatnie położenie robota"=w422, "Mapa z wprowadzonym punktem"=w428) -> ("Przesunięcie wycentrowane"=w426:T5)  [unwired: 9 in]
        n162 = property on="Mapa" class="Pict"("ZoomFactor"="Zoom mapy") -> ()  [unwired: 2 in, 2 out]
        n163 = Bundle By Name(cluster=w424, "Przesunięcie mapy"=w426, "Zoom"="Zoom mapy") -> (w425:T6)
      }
      event "Położenie startu": Value Change {
        n164 = event-data() -> ()  [unwired: 1 in, 5 out]
        n165 = Unbundle By Name(w435) -> ("Poł. startowe"=w433:cluster{"Piksel x":i32, "Piksel y":i32})
        n166 = control-ref of="Mapa"() -> (w432:refnum<vi>)
        n167 = call "Centrowanie położenia.vi"("Ostatnie położenie robota"=w433, "Mapa z wprowadzonym punktem"=w432) -> ("Przesunięcie wycentrowane"=w431:T5)  [unwired: 9 in]
        n168 = Bundle By Name(cluster=w434, "Przesunięcie mapy"=w431) -> (w436:T6)
      }
      event "stop": Value Change {
        n169 = event-data() -> ()  [unwired: 1 in, 5 out]
        n170 = Send Notification(notification="stop", notifier=w440) -> ()  [unwired: 1 in, 2 out]
      }
      event "Mapa": Mouse Down {
        # "Odczyt lokalizacji kursora po kliknięciu na mapie."
        n171 = event-data() -> ()  [unwired: 1 in, 2 out]
        n172 = property on="Mapa" class="Pict"() -> ("Mouse"=w452:T28)  [unwired: 2 in, 2 out]
        n173 = Unbundle By Name(w447) -> ("Przesunięcie mapy"=w446:cluster{"X":i16, "Y":i16})
        n174 = Unbundle By Name(w452) -> ("Mouse Position"=w449:cluster{"X":i32, "Y":i32})
        n175 = case shown="False" "Blokada \nznaczników" {
          tunnel: w449 -> [w454 _]
          tunnel: w446 -> [w453 _]
          frame False {
            n176 = Subtract(x=w454, y=w453) -> (x-y=w455:cluster{"X":i32, "Y":i32})
            n177 = case shown="True" "Wybór \nznacznika" {
              tunnel: w455 -> [w457 w458]
              frame False {
                n178 = local write "Polozenie 1"(w457) -> ()
              }
              frame True {
                n179 = local write "Polozenie 2"(w458) -> ()
              }
            }
          }
          frame True {
          }
        }
        n180 = local write "Mouse down coords"(w449) -> ()
      }
      event "Mapa": Mouse Up {
        # "Wyznaczenie zmiany położenia przed i po kliknięciu."
        n181 = event-data() -> ()  [unwired: 1 in, 7 out]
        n182 = property on="Mapa" class="Pict"() -> ("Mouse"=w482:T28)  [unwired: 2 in, 2 out]
        n183 = Unbundle By Name(w482) -> ("Mouse Position"=w477:cluster{"X":i32, "Y":i32})
        n184 = Unbundle By Name(w461) -> ("Przesunięcie mapy"=w464:cluster{"X":i16, "Y":i16})
        n185 = Subtract(x=w477, y="Mouse down coords") -> (x-y=w481:T5)
        n186 = Add(x=w481, y=w464) -> (x+y=w463:T5)
        n187 = Unbundle By Name(w461) -> ("Długość piksela w metrach"=w460:dbl)
        n188 = Subtract(x=w477, y=w463) -> (x-y=w476:T5)
        n189 = local read "Pocz. poł. \nrobota"() -> (w465:T1)
        n190 = local write "Ostatni zaznaczony punkt na mapie"(w476) -> ()
        n191 = Unbundle By Name(w465) -> ("Poł. startowe.Piksel x"=w474:i32, "Poł. startowe.Piksel y"=w473:i32)
        n192 = Unbundle By Name(w476) -> ("Horizontal"=w475:i32, "Vertical"=w472:i32)
        n193 = Subtract(x=w475, y=w474) -> (x-y=w470:i32)
        n194 = Subtract(x=w473, y=w472) -> (x-y=w471:i32)
        n195 = Multiply(x=w460, y=w470) -> (x*y=w467:dbl)
        n196 = Multiply(x=w460, y=w471) -> (x*y=w466:dbl)
        n197 = Bundle By Name(cluster=w461, "Przesunięcie mapy"=w463) -> (w462:T6)
        n198 = Bundle By Name(cluster=cluster{"X":dbl, "Y":dbl} {"X"=0.0, "Y"=10.497940558495968} ("Odleglosc do\n zaznaczonego punktu [m]"), "X"=w467, "Y"=w466) -> (w468:cluster{"X":dbl, "Y":dbl})
        n199 = local write "Odleglosc do\n zaznaczonego punktu [m]"(w468) -> ()
      }
      event "Odleglosc do\n zaznaczonego punktu [m]": Value Change {
        n200 = event-data() -> ()  [unwired: 1 in, 5 out]
        n201 = local read "Odleglosc do\n zaznaczonego punktu [m]"() -> (w498:cluster{"X":dbl, "Y":dbl})
        n202 = Unbundle By Name(w495) -> ("Długość piksela w metrach"=w494:dbl)
        n203 = local read "Pocz. poł. \nrobota"() -> (w490:T1)
        n204 = Unbundle By Name(w498) -> ("X"=w491:dbl, "Y"=w493:dbl)
        n205 = Unbundle By Name(w490) -> ("Poł. startowe.Piksel x"=w488:i32, "Poł. startowe.Piksel y"=w489:i32)
        n206 = Negate(x=w493) -> (-x=w492:dbl)
        n207 = Divide(x=w492, y=w494) -> (x/y=w486:dbl)
        n208 = Divide(x=w491, y=w494) -> (x/y=w487:dbl)
        n209 = Add(x=w487, y=w488) -> (x+y=w485:dbl)
        n210 = Add(x=w486, y=w489) -> (x+y=w484:dbl)
        n211 = Bundle By Name(cluster=cluster{"X":i32, "Y":i32} {"X"=0, "Y"=0} ("Ostatni zaznaczony punkt na mapie"), "X"=w485, "Y"=w484) -> (w497:cluster{"X":i32, "Y":i32})
        n212 = local write "Ostatni zaznaczony punkt na mapie"(w497) -> ()
      }
      event "Dodaj punkt wsp.": Value Change {
        n213 = event-data() -> ()  [unwired: 1 in, 5 out]
        n214 = local read "Pocz. poł. \nrobota"() -> (w506:T1)
        n215 = Unbundle By Name(w506) -> ("UTM"=w505:T4)
        n216 = call "Dodanie punktu do listy punkty na podstawie współrzędnych geograficznych.vi"("Nazwa punktu"="Nazwa", "UTM"=w505, "Współrzędne punktu"="Współrzędna punktu", "Lista współrzędnych"=w509) -> ("output array"=w502:string[][])  [unwired: 7 in]
        n217 = control-ref of="Kierunek na punkt"() -> (w504:refnum<vi>)
        n218 = control-ref of="Punkt do usunięcia"() -> (w503:refnum<vi>)
        n219 = call "Aktualizacja listy z punktami do usunięcia.vi"("Lista współrzędnych"=w502, "Lista z punktami do usunięcia"=w503) -> ()  [unwired: 10 in]
        n220 = call "Aktualizacja listy z punktami do usunięcia.vi"("Lista współrzędnych"=w502, "Lista z punktami do usunięcia"=w504) -> ()  [unwired: 10 in]
      }
    }
  }
  n221 = Destroy User Event(user event=w18) -> ()  [unwired: 1 in, 1 out]
  n222 = Unregister For Events(event registration refnum=w19) -> ()  [unwired: 1 in, 1 out]
